vi "Refresh Labels.vi"(4 "channel":T2, 6 "Lbl by name?":bool, 7 "Label":string, 8 "error in":errorcluster, 11 "Item Ref":T1 format="%.0x") -> (0 "error out":errorcluster)   [LabVIEW 2012, in "AIT 429 System Explorer.lvlib"]
uses:
  AIT 429 System Explorer.lvlib
  Controls/AIT_Channel.ctl
  Controls/AIT_Label.ctl
  Controls/AIT_Word.ctl
  Controls/ARINCParam.ctl
  Shared/Controls and Global/TransferType.ctl
  <userlib>/ARINC-429/vi/enum/Owl429ChannelSpeed.ctl
  <vilib>/NI Veristand/Custom Device API/Custom Device Item Ref.ctl
  Build Param Properties.vi
  Shared/Word to double.vi
  <vilib>/NI Veristand/Custom Device Tools/Custom Device Utility Library/NI VeriStand - Search for Item by Name.vi
  <vilib>/NI Veristand/Custom Device Tools/Custom Device Utility Library/NI VeriStand - Search for All Items by Property.vi
  <vilib>/NI Veristand/Custom Device API/Get Item Property (U32).vi
  <vilib>/NI Veristand/Custom Device API/Get Item Property (Boolean).vi
  Shared/Controls and Global/Global.vi
  <vilib>/NI Veristand/Custom Device API/NI VeriStand - Add Custom Device Section.vi
  AddParamChannels.vi
  <vilib>/NI Veristand/Custom Device API/NI VeriStand - Add Custom Device Channel.vi
  <vilib>/NI Veristand/Custom Device API/Set Item Property (Variant).vi
  <vilib>/NI Veristand/Custom Device Tools/Custom Device Utility Library/NI VeriStand - Search for All Items by GUID.vi
  <vilib>/NI Veristand/Custom Device API/NI VeriStand - Get Item GUID.vi
  <vilib>/NI Veristand/Custom Device API/NI VeriStand - Get Item Parent.vi
  <vilib>/NI Veristand/Custom Device API/NI VeriStand - Set Custom Device Channel Default Value.vi
  <vilib>/NI Veristand/Custom Device API/Get Item Property (Double).vi
  <vilib>/NI Veristand/Custom Device API/Get Item Property (I32).vi
  <vilib>/NI Veristand/Custom Device Tools/Custom Device Utility Library/Custom Device Utility Library.lvlib
  <vilib>/NI Veristand/Custom Device API/Custom Device API.lvlib
  ARINC 429 Shared.lvlib
  <userlib>/ARINC-429/Owl429.lvlib
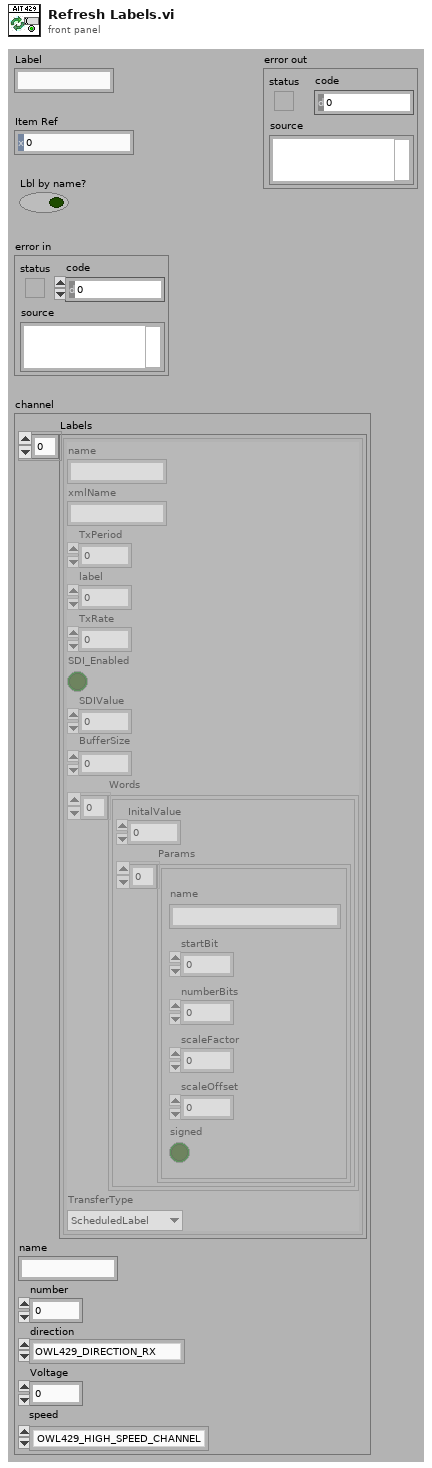
[diagram p1: front panel]
types:
  T1 = typedef "Custom Device API.lvlib/Custom Device Item Ref.ctl" = u64
  T2 = typedef "AIT 429 System Explorer.lvlib/AIT_Channel.ctl" = cluster{"Labels":T3[], "name":string, "number":u8, "direction":enum16{"OWL429_DIRECTION_RX", "OWL429_DIRECTION_TX"}, "Voltage":dbl, "speed":T7}
  T3 = typedef "AIT 429 System Explorer.lvlib/AIT_Label.ctl" = cluster{"name":string, "xmlName":string, "TxPeriod":u32, "label":u32, "TxRate":dbl, "SDI_Enabled":bool, "SDIValue":u8, "BufferSize":u32, "Words":T4[], "TransferType":T6}
  T4 = typedef "AIT 429 System Explorer.lvlib/AIT_Word.ctl" = cluster{"InitalValue":u32, "Params":T5[]}
  T5 = typedef "AIT 429 System Explorer.lvlib/ARINCParam.ctl" = cluster{"name":string, "startBit":i32, "numberBits":i32, "scaleFactor":dbl, "scaleOffset":dbl, "signed":bool}
  T6 = typedef "ARINC 429 Shared.lvlib/TransferType.ctl" = enum16{"ScheduledLabel", "Acyclic", "Block", "Strobe"}
  T7 = typedef "Owl429.lvlib/Owl429ChannelSpeed.ctl" = enum16{"OWL429_HIGH_SPEED_CHANNEL", "OWL429_LOW_SPEED_CHANNEL"}
  T8 = enum16{"OWL429_DIRECTION_RX", "OWL429_DIRECTION_TX"}
  T9 = typedef "Custom Device API.lvlib/Custom Device Item Info.ctl" = cluster{"Name":string, "Is Channel":bool, "GUID":string, "Is Waveform":bool}
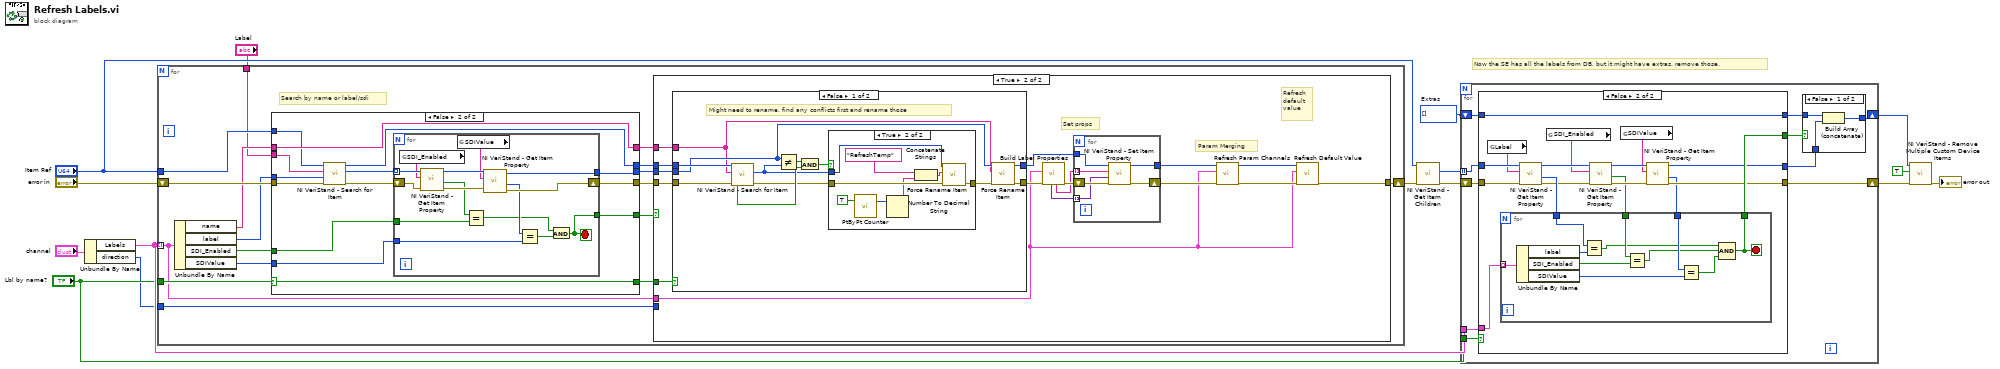
[diagram p0: block diagram]
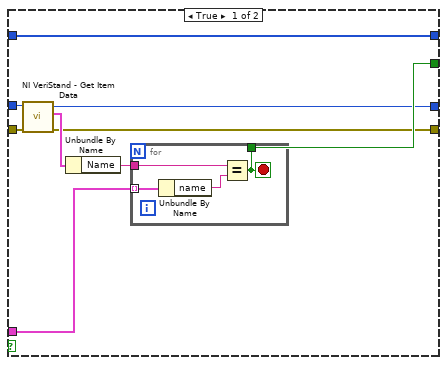
[diagram p3: hidden frame]
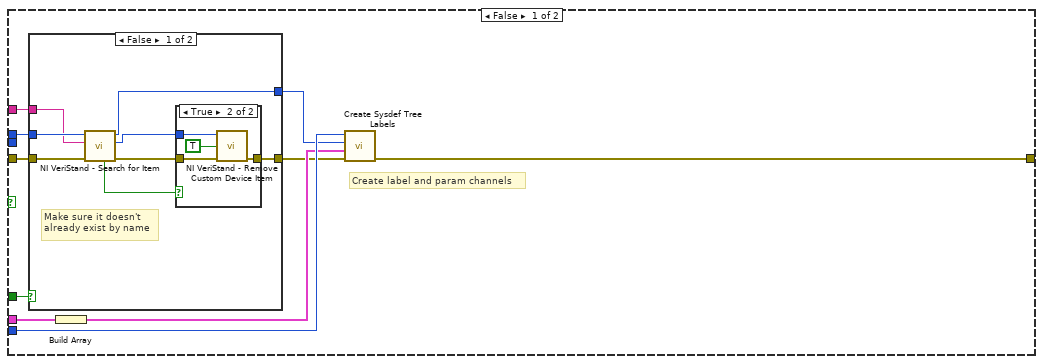
[diagram p4: hidden frame]
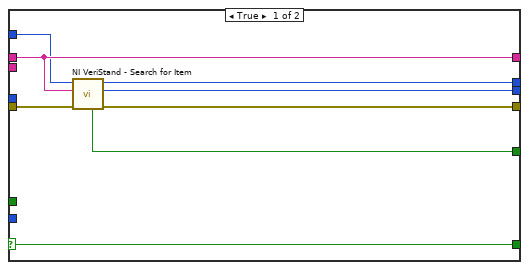
[diagram p9: hidden frame]
diagram:
  w12 = T1[] []  # Extras
  # "Now the SE has all the labels from DB, but it might have extras, remove those."
  n1 = Unbundle By Name("channel") -> ("Labels"=w11:T3[], "direction"=w4:T8)
  n2 = for {
    shift-right: [w21] -> w5
    shift-left: "error in" -> [w32]
    tunnel: w11 -> [w19] mode=indexing
    tunnel: "Lbl by name?" -> [w31]
    tunnel: "Item Ref" -> [w29]
    tunnel: "Label" -> [w27]
    tunnel: w4 -> [w20]
    # "Search by name or label/sdi"
    n3 = Unbundle By Name(w19) -> ("name"=w30:string, "label"=w28:u32, "SDI_Enabled"=w17:bool, "SDIValue"=w16:u8)
    n4 = case shown="False" w31 {
      selector: w31 -> [w104 w119]
      tunnel: w32 -> [w110 w124]
      tunnel: w30 -> [w105 w120]
      tunnel: w29 -> [w103 w118]
      tunnel: [w109 w112] -> w26
      tunnel: [w108 w113] -> w24
      tunnel: [w107 w111] -> w18
      tunnel: w27 -> [_ w123]
      tunnel: w28 -> [_ w122]
      tunnel: [w106 w121] -> w22
      tunnel: [w105 w120] -> w23
      tunnel: [w104 w119] -> w25
      tunnel: w17 -> [_ w115]
      tunnel: w16 -> [_ w114]
      frame True {
        n5 = call-poly <vilib>:"NI VeriStand - Search for Item.vi"("error in"=w110, "Item Name"=w105, "Section Ref in"=w103) -> ("error out"=w108:errorcluster, "Item Ref"=w107:T1, "Section Ref out"=w106:T1, "Found"=w109:bool)  [unwired: 5 in]
      }
      frame False {
        n6 = call-poly <vilib>:"NI VeriStand - Search for Item.vi"("error in"=w124, "Property Value"=w122, "Property Name"=w123, "Section Ref in"=w118) -> ("error out"=w117:errorcluster, "Item Refs"=w116:T1[], "Section Ref out"=w121:T1)  [unwired: 4 in, 1 out]
        n7 = for {
          tunnel: w116 -> [w138] mode=indexing
          tunnel: w115 -> [w131]
          tunnel: w114 -> [w129]
          shift-right: [w133] -> w113
          shift-left: w117 -> [w139]
          tunnel: [w126] -> w112
          tunnel: [w125] -> w111
          stop <- w126 stop-if-true
          n8 = global read "Global.vi" "SDI_Enabled"() -> (w137:string)
          n9 = call-poly <vilib>:"NI VeriStand - Get Item Property.vi"("error in (no error)"=w139, "Property Name"=w137, "Item Ref in"=w138) -> ("error out"=w134:errorcluster, "Value"=w132:bool, "Item Ref out"=w136:T1)  [unwired: 5 in, 1 out]
          n10 = global read "Global.vi" "SDIValue"() -> (w135:string)
          n11 = Equal?(x=w132, y=w131) -> (x = y?=w127:bool)
          n12 = call-poly <vilib>:"NI VeriStand - Get Item Property.vi"("error in (no error)"=w134, "Property Name"=w135, "Item Ref in"=w136) -> ("error out"=w133:errorcluster, "Value"=w130:u32, "Item Ref out"=w125:T1)  [unwired: 5 in, 1 out]
          n13 = Equal?(x=w130, y=w129) -> (x = y?=w128:bool)
          n14 = And(x=w127, y=w128) -> (x .and. y?=w126:bool)
        }
      }
    }
    n15 = case shown="True" w26 {
      tunnel: w25 -> [w42 w73]
      tunnel: w24 -> [w41 w72]
      tunnel: w23 -> [w40 w63]
      tunnel: w22 -> [w39 w70]
      tunnel: [w34 w64] -> w21
      tunnel: w19 -> [w36 w58]
      tunnel: w20 -> [w38 _]
      tunnel: w18 -> [_ w71]
      frame False {
        # "Create label and param channels"
        n16 = case shown="False" w42 {
          tunnel: w41 -> [w50 w57]
          tunnel: w39 -> [w49 w56]
          tunnel: w40 -> [w44 _]
          tunnel: [w46 w57] -> w33
          tunnel: [w45 w56] -> w37
          frame False {
            # "Make sure it doesn't\nalready exist by name"
            n17 = call-poly <vilib>:"NI VeriStand - Search for Item.vi"("error in"=w50, "Item Name"=w44, "Section Ref in"=w49) -> ("error out"=w48:errorcluster, "Item Ref"=w47:T1, "Section Ref out"=w45:T1, "Found"=w43:bool)  [unwired: 5 in]
            n18 = case shown="True" w43 {
              tunnel: w48 -> [w51 w55]
              tunnel: w47 -> [_ w54]
              tunnel: [w51 w52] -> w46
              frame False {
              }
              frame True {
                n19 = call <vilib>:"NI VeriStand - Remove Custom Device Item.vi"("error in (no error)"=w55, "Force Delete (F)"=TRUE, "Item Ref in"=w54) -> ("error out"=w52:errorcluster)  [unwired: 7 in, 1 out]
              }
            }
          }
          frame True {
          }
        }
        n20 = Build Array(w36) -> (w35:T3[])
        n21 = call "Create Sysdef Tree Labels.vi"("error in"=w33, "Labels"=w35, "Section Ptr"=w37, "direction"=w38) -> ("error out"=w34:errorcluster)  [unwired: 7 in]
      }
      frame True {
        # "Refresh\ndefault\nvalue"
        # "Param Merging"
        # "Set props"
        n22 = case shown="False" w73 {
          tunnel: w72 -> [w90 w102]
          tunnel: w71 -> [w82 w101]
          tunnel: [w91 w102] -> w69
          tunnel: w70 -> [w89 _]
          tunnel: [w81 w101] -> w67
          tunnel: w63 -> [w80 _]
          frame False {
            # "Might need to rename, find any conflicts first and rename those"
            n23 = call-poly <vilib>:"NI VeriStand - Search for Item.vi"("error in"=w90, "Item Name"=w80, "Section Ref in"=w89) -> ("error out"=w85:errorcluster, "Item Ref"=w84:T1, "Found"=w87:bool)  [unwired: 5 in, 1 out]
            n24 = Not Equal?(x=w82, y=w84) -> (x != y?=w88:bool)
            n25 = And(x=w88, y=w87) -> (x .and. y?=w86:bool)
            n26 = case shown="True" w86 {
              tunnel: w85 -> [w92 w100]
              tunnel: w84 -> [_ w99]
              tunnel: [w92 w98] -> w83
              frame False {
              }
              frame True {
                n27 = call "PtByPt Counter.vi"("activate"=TRUE) -> ("counter"=w96:u32)  [unwired: 1 in, 1 out]
                n28 = Number To Decimal String(number=w96) -> (decimal integer string=w95:string)  [unwired: 1 in]
                n29 = Concatenate Strings("RefreshTemp", w95) -> (w93:string)
                n30 = call "Force Rename Item.vi"("error in"=w100, "String"=w93, "Item Ref"=w99) -> ("error out"=w98:errorcluster)  [unwired: 7 in, 1 out]
              }
            }
            n31 = call "Force Rename Item.vi"("error in"=w83, "String"=w80, "Item Ref"=w82) -> ("error out"=w91:errorcluster, "Item Ref out"=w81:T1)  [unwired: 7 in]
          }
          frame True {
            # "Item found by name, don't need to rename"
          }
        }
        n32 = call "Build Label Properties.vi"("error in (no error)"=w69, "Labels"=w58) -> ("error out"=w68:errorcluster, "Prop Names"=w66:string[], "Prop Values"=w65:variant[])  [unwired: 6 in, 1 out]
        n33 = for {
          shift-right: [w75] -> w62
          shift-left: w68 -> [w79]
          tunnel: w67 -> [w78]
          tunnel: w66 -> [w77] mode=indexing
          tunnel: w65 -> [w76] mode=indexing
          tunnel: [w74] -> w60
          n34 = call-poly <vilib>:"NI VeriStand - Set Item Property.vi"("error in (no error)"=w79, "Value"=w76, "Property Name"=w77, "Item Ref in"=w78) -> ("error out"=w75:errorcluster, "Item Ref out"=w74:T1)  [unwired: 5 in, 1 out]
        }
        n35 = call "Refresh Param Channels.vi"("error in (no error)"=w62, "Label"=w58, "Param Ref in"=w60) -> ("error out"=w61:errorcluster, "Param Ref out"=w59:T1)  [unwired: 7 in]
        n36 = call "Refresh Default Value.vi"("error in (no error)"=w61, "Label"=w58, "Param Ref in"=w59) -> ("error out"=w64:errorcluster)  [unwired: 7 in, 1 out]
      }
    }
  }
  n37 = call <vilib>:"NI VeriStand - Get Item Children.vi"("error in (no error)"=w5, "Item Ref in"="Item Ref") -> ("error out"=w7:errorcluster, "Child Refs"=w8:T1[])  [unwired: 6 in, 2 out]
  n38 = for {
    shift-right: [w145] -> w13
    shift-left: w7 -> [w149]
    tunnel: w8 -> [w148] mode=indexing
    tunnel: w11 -> [w146]
    tunnel: "Lbl by name?" -> [w147]
    shift-right: [w141] -> w14
    shift-left: w12 -> [w144]
    n39 = case shown="False" w147 {
      tunnel: w149 -> [w162 w183]
      tunnel: w148 -> [w161 w182]
      tunnel: w146 -> [w159 w181]
      tunnel: [w157 w180] -> w143
      tunnel: [w156 w171] -> w145
      tunnel: w144 -> [w155 w179]
      tunnel: [w155 w179] -> w142
      tunnel: [w154 w172] -> w140
      frame True {
        n40 = call <vilib>:"NI VeriStand - Get Item Data.vi"("error in (no error)"=w162, "Item Ref in"=w161) -> ("error out"=w156:errorcluster, "Item Info"=w160:T9, "Item Ref out"=w154:T1)  [unwired: 6 in, 1 out]
        n41 = Unbundle By Name(w160) -> ("Name"=w158:string)
        n42 = for {
          tunnel: w159 -> [w166] mode=indexing
          tunnel: w158 -> [w164]
          tunnel: [w163] -> w157
          stop <- w163 stop-if-true
          n43 = Unbundle By Name(w166) -> ("name"=w165:string)
          n44 = Equal?(x=w164, y=w165) -> (x = y?=w163:bool)
        }
      }
      frame False {
        n45 = global read "Global.vi" "Label"() -> (w178:string)
        n46 = call-poly <vilib>:"NI VeriStand - Get Item Property.vi"("error in (no error)"=w183, "Property Name"=w178, "Item Ref in"=w182) -> ("error out"=w176:errorcluster, "Value"=w177:u32, "Item Ref out"=w175:T1)  [unwired: 5 in, 1 out]
        n47 = global read "Global.vi" "SDI_Enabled"() -> (w170:string)
        n48 = call-poly <vilib>:"NI VeriStand - Get Item Property.vi"("error in (no error)"=w176, "Property Name"=w170, "Item Ref in"=w175) -> ("error out"=w173:errorcluster, "Value"=w168:bool, "Item Ref out"=w174:T1)  [unwired: 5 in, 1 out]
        n49 = global read "Global.vi" "SDIValue"() -> (w169:string)
        n50 = call-poly <vilib>:"NI VeriStand - Get Item Property.vi"("error in (no error)"=w173, "Property Name"=w169, "Item Ref in"=w174) -> ("error out"=w171:errorcluster, "Value"=w167:u32, "Item Ref out"=w172:T1)  [unwired: 5 in, 1 out]
        n51 = for {
          tunnel: w181 -> [w194] mode=indexing
          tunnel: w177 -> [w192]
          tunnel: [w184] -> w180
          tunnel: w168 -> [w191]
          tunnel: w167 -> [w188]
          stop <- w184 stop-if-true
          n52 = Unbundle By Name(w194) -> ("label"=w193:u32, "SDI_Enabled"=w190:bool, "SDIValue"=w189:u8)
          n53 = Equal?(x=w192, y=w193) -> (x = y?=w187:bool)
          n54 = Equal?(x=w191, y=w190) -> (x = y?=w186:bool)
          n55 = Equal?(x=w188, y=w189) -> (x = y?=w185:bool)
          n56 = Compound Arithmetic op=AND(w187, w186, w185) -> (w184:bool)
        }
      }
    }
    n57 = case shown="False" w143 {
      tunnel: w142 -> [w152 w153]
      tunnel: [w151 w153] -> w141
      tunnel: w140 -> [w150 _]
      frame False {
        n58 = Build Array (concatenate)(w152, w150) -> (w151:T1[])
      }
      frame True {
      }
    }
  }
  n59 = call <vilib>:"NI VeriStand - Remove Multiple Custom Device Items.vi"("error in (no error)"=w13, "Force Delete (F)"=TRUE, "Item Refs in"=w14) -> ("error out"=→"error out":errorcluster)  [unwired: 7 in, 1 out]
